vi "全局变量1.vi"() -> ()   [LabVIEW 2023]
panel:
  out "while开关":bool
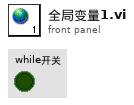
[diagram p1: front panel]
diagram:
